vi "Signal Error.vi"(3 "DO Task":refnum<k21>="BlueSimple_DO", 4 "Error bong?":bool=TRUE) -> ()   [LabVIEW 2010]
uses:
  Controls/Bits to Write.ctl
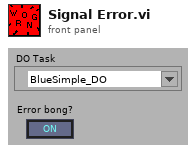
[diagram p1: front panel]
types:
  T1 = typedef "Bits to Write.ctl" = enum16{"LED 1 on", "LED 1 off", "LED 2 on", "LED 2 off", "LED 3 on", "LED 3 off", "LED 4 on", "LED 4 off", "All LEDs on", "All LEDs off", "In trial on", "In trial off", "Buzzer on", "Buzzer off", "Reward on", "Reward off", "Target number", "Trial type preQ on", "Trial type preQ off", "Error on", "Error off", "Trial number", "DBS on", "DBS off", "Sine on", "Sine off", "All Bits On", "All Bits Off", "Init", "Specify mask/pattern"}
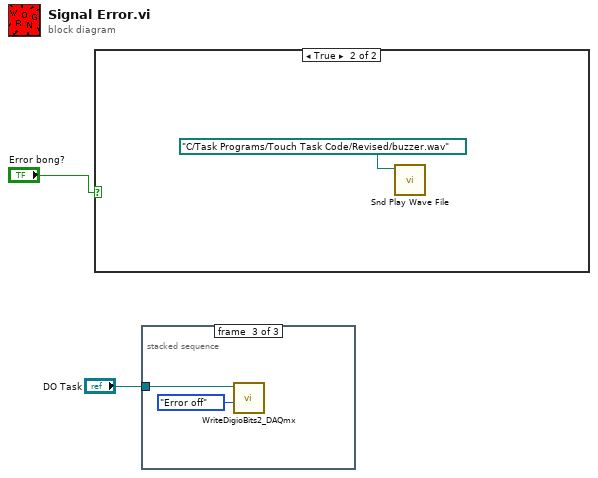
[diagram p0: block diagram]
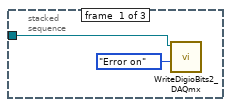
[diagram p2: hidden frame]
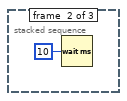
[diagram p3: hidden frame]
diagram:
  n1 = case shown="True" "Error bong?" {
    frame False {
    }
    frame True {
      n2 = call <vilib>:"Snd Play Wave File.vi"("wave file path"=path "C:/Task Programs/Touch Task Code/Revised/buzzer.wav") -> ()  [unwired: 9 in, 2 out]
    }
  }
  n3 = stacked-sequence {
    tunnel: "DO Task" -> [w4 _ w8]
    frame #0 {
      n4 = call "WriteDigioBits2_DAQmx.vi"("Bits to write"=Bits_to_Write."Error on", "DO Task"=w4) -> ()  [unwired: 9 in, 1 out]
    }
    frame #1 {
      n5 = Wait (ms)(milliseconds to wait=u32 10) -> ()  [unwired: 1 out]
    }
    frame #2 {
      n6 = call "WriteDigioBits2_DAQmx.vi"("Bits to write"=Bits_to_Write."Error off", "DO Task"=w8) -> ()  [unwired: 9 in, 1 out]
    }
  }
